vi "FTW-WebService-IncomingRequestRouter.vi"(9 "RequestURI":string caption="This special input is set directly by ws_runtime.dll,\nbut only because we have specifically defined\n\"RequestURI\" as the token to be populated based\non the routing rules in WebService.ini.", 10 "httpRequestID":u32 caption="This special input is set directly by ws_runtime.dll", 11 "NI_wsHandle":u32 caption="This special input is set directly by ws_runtime.dll") -> ()   [LabVIEW 2015, in "FTW-WebService.lvclass"]
uses:
  FTW-WebService.lvclass
panel:
  in  "Application Messenger":refnum<user-event> caption="This input is set by the InitializeRouter method of this class\nvia a Set Control Value method -- do not change the name!"
  in  "Timeout":i32=2500 caption="This input is set by the InitializeRouter method of this class\nvia a Set Control Value method -- do not change the name!" format="%dmsec"
  # "Inputs set by Web Service Callback Framework"
  # "Inputs set once dynamically during application launch"
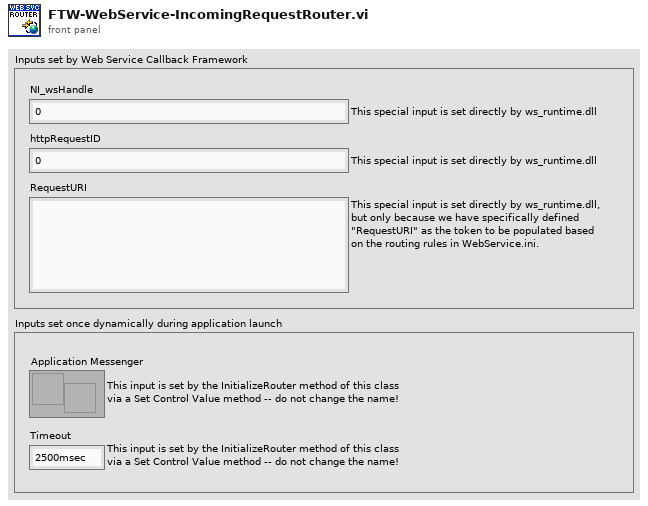
[diagram p1: front panel]
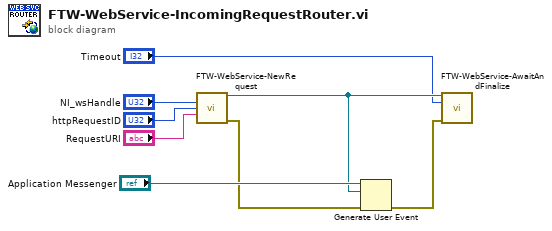
[diagram p0: block diagram]
diagram:
  n1 = call "FTW-WebService-NewRequest.vi"("NI_wsHandle"="NI_wsHandle", "httpRequestID"="httpRequestID", "RequestURI"="RequestURI") -> ("FTW Web Request"=w5:refnum<class "FTW-WebService.lvclass">, "error out"=w7:errorcluster)  [unwired: 11 in]
  n2 = Generate User Event(user event="Application Messenger", event data cluster=w5, error in=w7) -> (error out=w6:errorcluster)  [unwired: 1 in, 1 out]
  n3 = call "FTW-WebService-AwaitAndFinalize.vi"("FTW Web Request"=w5, "Timeout"="Timeout", "error in"=w6) -> ()  [unwired: 12 in, 1 out]
